vi "InitializeFileNoDig.vi"(0 "File Path":path=path "C:/Users/lbignell/Desktop/1 Ton Tank Experiment/Control Software/HDF5/Dummy2.h5", 1 "Thermocouple Location":string[](array[string])=["In Dark Box", "In Room"], 2 "Run Number":i32, 3 "VME Configuration":T1={"Module Description"=["Bridge", "TDC", "Scaler", "Hodoscope QDC ", "Other QDC", "Digitizer 1", "Digitizer 2", ""], "Module Model"=["V2718", "V775", "V830", "V965A", "V965A", "V1729A", "1729A", ""], "Module Address"=[0, 4026597376, 4026662912, 4026728448, 4026793984, 4026859520, 4026925056]} {"Module Address" format="%.0x"}, 4 "Trigger Bit Descriptions":string[](array[string])=["TrigA", "TrigB", "TrigC", "TrigD"], 5 "error in":errorcluster, 6 "Scaler Info":T3={"Chanel Description"=["H0", "H1", "H2", "H3", "H4", "H5", "TrigA", "TrigB", "TrigC", "TrigD", "Ch0", "Ch1", "Ch2", "Ch3", "Ch4", "Ch5", "Ch6", "Ch7"], "Only Hodo?"=[TRUE, TRUE, TRUE, TRUE, TRUE, TRUE, TRUE, TRUE, FALSE, FALSE, FALSE, FALSE, FALSE, FALSE, FALSE, FALSE, FALSE, FALSE]}, 7 "Optional Comments":string, 9 "Material in Tank":string(combo), 10 "Run Type":string(combo), 11 "TDC Info":T3={"Chanel Description"=["H0", "H1", "H2", "H3", "H4", "H5", "TrigA", "TrigB", "TrigC", "TrigD"], "Only Hodo?"=[TRUE, TRUE, TRUE, TRUE, TRUE, TRUE, TRUE, TRUE, FALSE, FALSE]}, 12 "QDC Info":T3={"Chanel Description"=["H0", "H1", "H2", "H3", "H4", "H5"], "Only Hodo?"=[TRUE, TRUE, TRUE, TRUE, TRUE, TRUE]}) -> (14 "File Handle":T2=16777216 format="%.0x", 19 "error out":errorcluster)   [LabVIEW 2014]
uses:
  <vilib>/addons/h5labview2/base/hid_t.ctl
  <vilib>/addons/h5labview2/file/H5Fmode.ctl
  <vilib>/addons/h5labview2/base/lib_path.vi
  <vilib>/addons/h5labview2/base/H5Equery.vi
  DatasetNames.vi
  <vilib>/addons/h5labview2/dataset/H5Dwrite.llb/H5Dwrite.xnode
  <vilib>/addons/h5labview2/file/H5F.lvlib
  <vilib>/addons/h5labview2/group/H5G.lvlib
  <vilib>/addons/h5labview2/props/H5P.lvlib
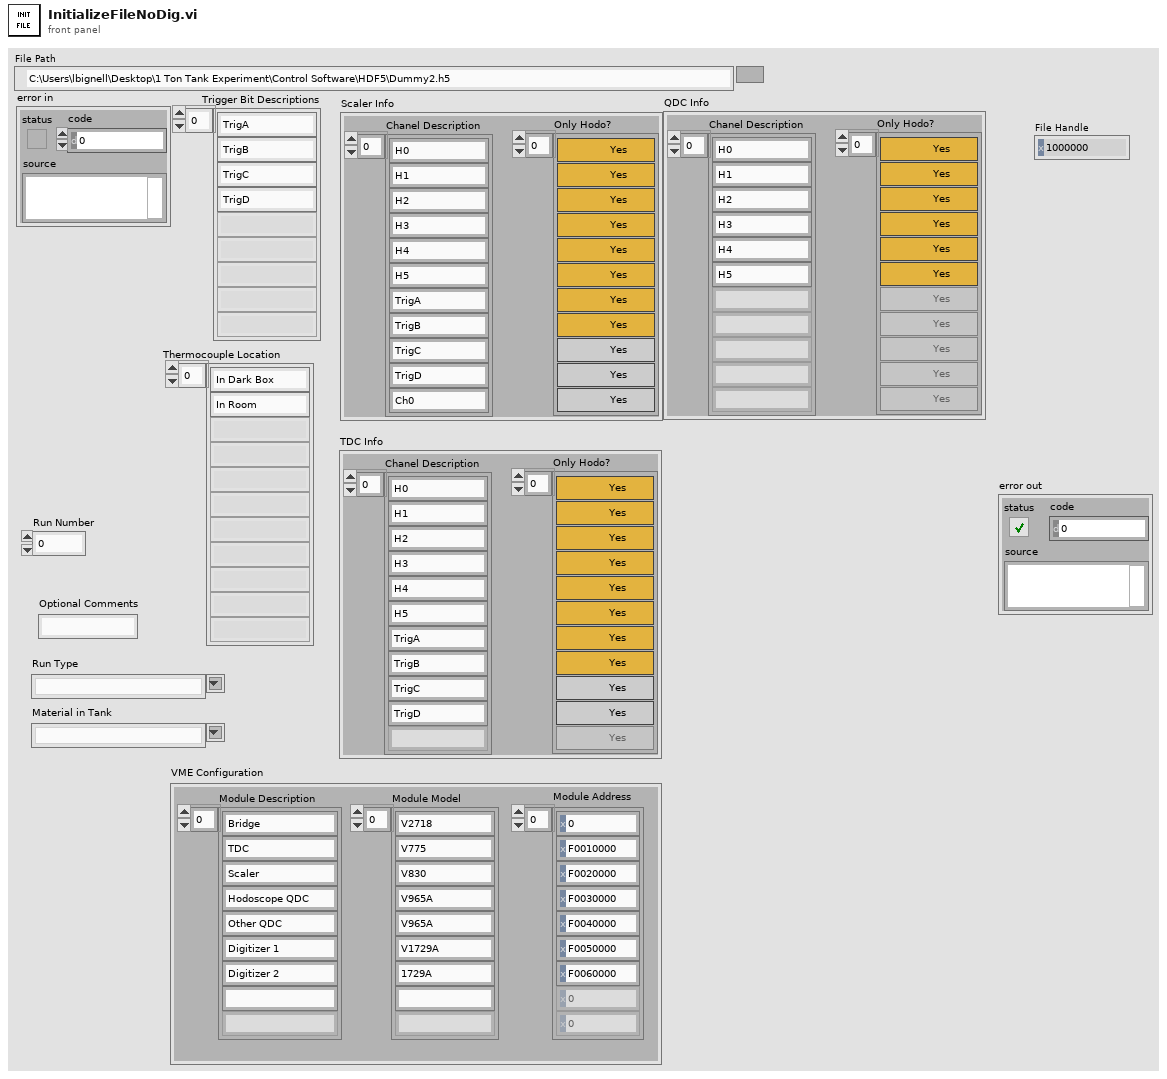
[diagram p1: front panel]
types:
  T1 = cluster{"Module Description":string[], "Module Model":string[], "Module Address":u32[]}
  T2 = typedef "hid_t.ctl" = i32
  T3 = cluster{"Chanel Description":string[], "Only Hodo?":bool[]}
  T4 = typedef "H5F.lvlib/H5Fmode.ctl" = enum16{"read-only", "read-write", "overwrite", "create new", "open or create"}
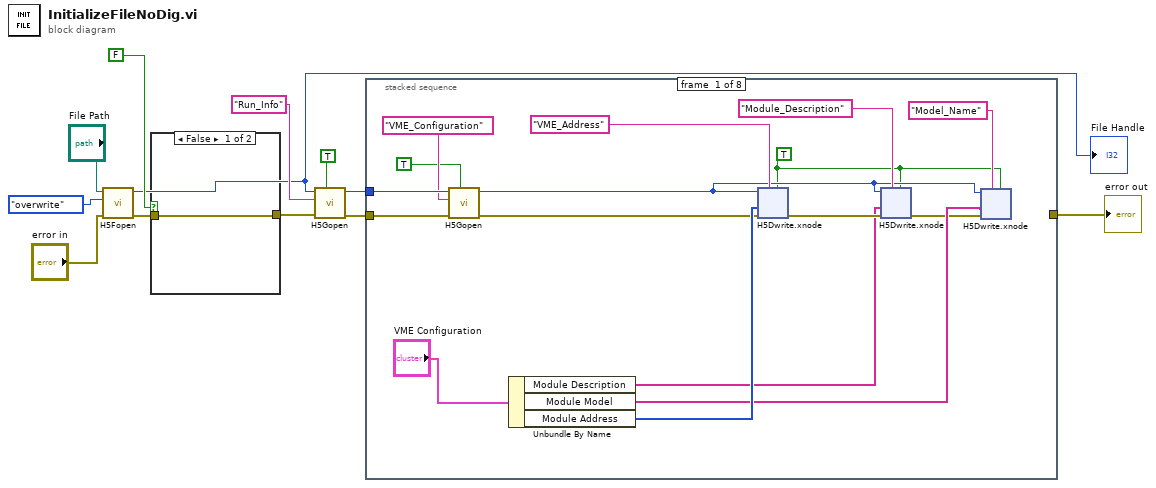
[diagram p0: block diagram]
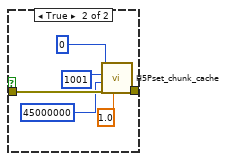
[diagram p2: hidden frame]
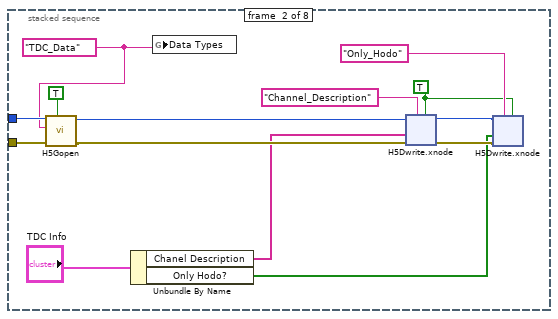
[diagram p3: hidden frame]
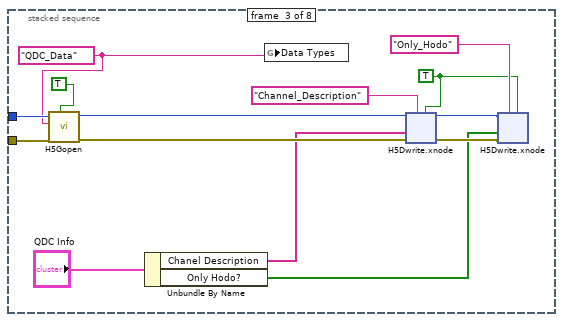
[diagram p4: hidden frame]
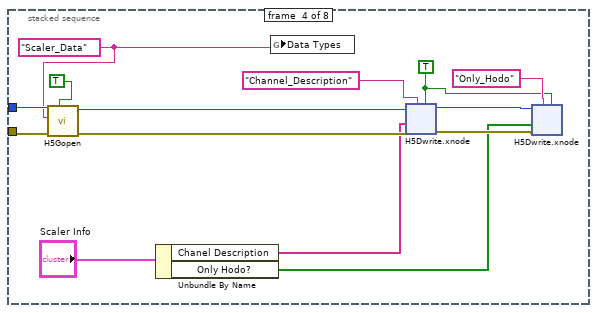
[diagram p5: hidden frame]
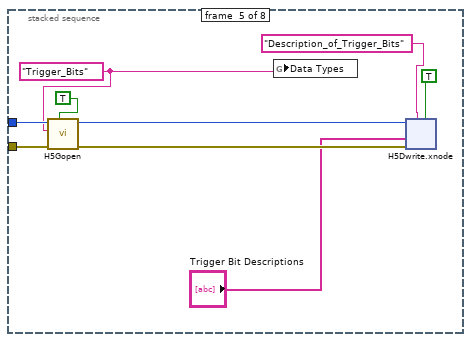
[diagram p6: hidden frame]
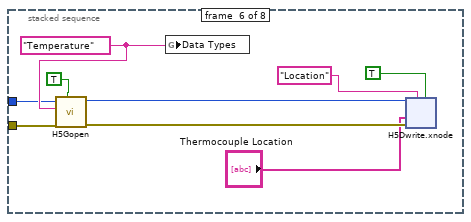
[diagram p7: hidden frame]
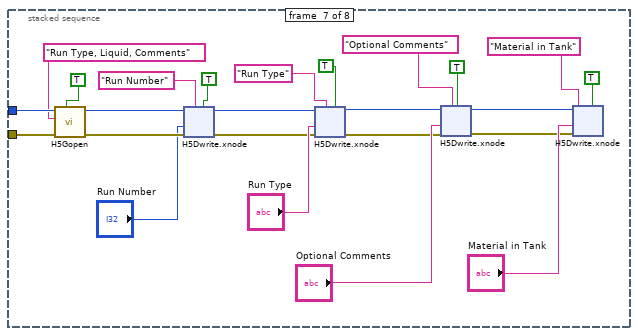
[diagram p8: hidden frame]
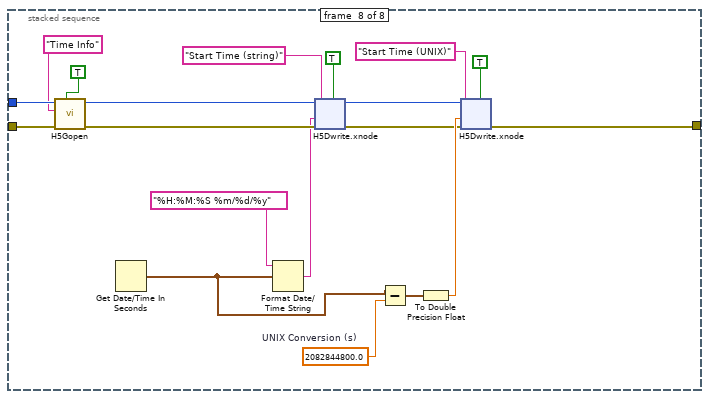
[diagram p9: hidden frame]
diagram:
  n1 = call <vilib>:"H5Fopen.vi"("error in (no error)"="error in", "mode (read-only)"=H5Fmode."overwrite", "path"="File Path") -> ("error out"=w4:errorcluster, "ref out"=w1:T2)  [unwired: 7 in]
  "File Handle" <- w1
  n2 = case shown="False" FALSE {
    tunnel: w4 -> [w13 w19]
    tunnel: [w13 w18] -> w3
    frame False {
    }
    frame True {
      n3 = call <vilib>:"H5Pset_chunk_cache.vi"("w0"=1.0, "error in (no error)"=w19, "nbytes"=u32 45000000, "nslots"=u32 1001, "prop in"=T2 0) -> ("error out"=w18:errorcluster)  [unwired: 5 in, 1 out]
    }
  }
  n4 = call <vilib>:"H5Gopen.vi"("create? (F)"=TRUE, "error in (no error)"=w3, "name"="Run_Info", "ref in"=w1) -> ("error out"=w7:errorcluster, "group out"=w8:T2)  [unwired: 6 in]
  n5 = stacked-sequence {
    tunnel: w8 -> [w31 w100 w151 w201 w247 w268 w316 w407]
    tunnel: w7 -> [w32 w102 w152 w202 w246 w274 w317 w408]
    tunnel: [_ _ _ _ _ _ _ w390] -> w6
    frame #0 {
      w21 = TRUE ("replace? (F)")
      n6 = call <vilib>:"H5Gopen.vi"("create? (F)"=TRUE, "error in (no error)"=w32, "name"="VME_Configuration" ("attrib name"), "ref in"=w31) -> ("error out"=w29:errorcluster, "group out"=w25:T2)  [unwired: 6 in]
      n7 = Unbundle By Name("VME Configuration") -> ("Module Description"=w26:string[], "Module Model"=w23:string[], "Module Address"=w33:u32[])
      n8 = xnode "H5Dwrite.xnode"("replace? (F)"=w21, "dataset name"="VME_Address" ("attrib name"), "error in (no error)"=w29, "data"=w33, "ref in"=w25) -> ("error out"=w27:errorcluster)  [unwired: 2 in, 2 out]
      n9 = xnode "H5Dwrite.xnode"("replace? (F)"=w21, "dataset name"="Module_Description" ("attrib name"), "error in (no error)"=w27, "data"=w26, "ref in"=w25) -> ("error out"=w22:errorcluster)  [unwired: 2 in, 2 out]
      n10 = xnode "H5Dwrite.xnode"("replace? (F)"=w21, "dataset name"="Model_Name" ("attrib name"), "error in (no error)"=w22, "data"=w23, "ref in"=w25) -> ()  [unwired: 2 in, 3 out]
    }
    frame #1 {
      w91 = TRUE ("replace? (F)")
      w99 = "TDC_Data" ("Combo Box")
      n11 = call <vilib>:"H5Gopen.vi"("create? (F)"=TRUE, "error in (no error)"=w102, "name"=w99, "ref in"=w100) -> ("error out"=w101:errorcluster, "group out"=w96:T2)  [unwired: 6 in]
      n12 = Unbundle By Name("TDC Info") -> ("Chanel Description"=w95:string[], "Only Hodo?"=w90:bool[])
      n13 = global write "DatasetNames.vi" "Data Types"(w99) -> ()
      n14 = xnode "H5Dwrite.xnode"("replace? (F)"=w91, "dataset name"="Channel_Description" ("attrib name"), "error in (no error)"=w101, "data"=w95, "ref in"=w96) -> ("error out"=w94:errorcluster, "ref out"=w93:i32)  [unwired: 2 in, 1 out]
      n15 = xnode "H5Dwrite.xnode"("replace? (F)"=w91, "dataset name"="Only_Hodo" ("attrib name"), "error in (no error)"=w94, "data"=w90, "ref in"=w93) -> ()  [unwired: 2 in, 3 out]
    }
    frame #2 {
      w141 = TRUE ("replace? (F)")
      w148 = "QDC_Data" ("Combo Box")
      n16 = call <vilib>:"H5Gopen.vi"("create? (F)"=TRUE ("replace? (F)"), "error in (no error)"=w152, "name"=w148, "ref in"=w151) -> ("error out"=w149:errorcluster, "group out"=w150:T2)  [unwired: 6 in]
      n17 = Unbundle By Name("QDC Info") -> ("Chanel Description"=w145:string[], "Only Hodo?"=w140:bool[])
      n18 = global write "DatasetNames.vi" "Data Types"(w148) -> ()
      n19 = xnode "H5Dwrite.xnode"("replace? (F)"=w141, "dataset name"="Channel_Description" ("attrib name"), "error in (no error)"=w149, "data"=w145, "ref in"=w150) -> ("error out"=w144:errorcluster, "ref out"=w143:i32)  [unwired: 2 in, 1 out]
      n20 = xnode "H5Dwrite.xnode"("replace? (F)"=w141, "dataset name"="Only_Hodo" ("attrib name"), "error in (no error)"=w144, "data"=w140, "ref in"=w143) -> ()  [unwired: 2 in, 3 out]
    }
    frame #3 {
      w190 = TRUE ("replace? (F)")
      w198 = "Scaler_Data" ("Combo Box")
      n21 = call <vilib>:"H5Gopen.vi"("create? (F)"=TRUE, "error in (no error)"=w202, "name"=w198, "ref in"=w201) -> ("error out"=w199:errorcluster, "group out"=w200:T2)  [unwired: 6 in]
      n22 = Unbundle By Name("Scaler Info") -> ("Chanel Description"=w195:string[], "Only Hodo?"=w191:bool[])
      n23 = global write "DatasetNames.vi" "Data Types"(w198) -> ()
      n24 = xnode "H5Dwrite.xnode"("replace? (F)"=w190, "dataset name"="Channel_Description" ("attrib name"), "error in (no error)"=w199, "data"=w195, "ref in"=w200) -> ("error out"=w194:errorcluster, "ref out"=w193:i32)  [unwired: 2 in, 1 out]
      n25 = xnode "H5Dwrite.xnode"("replace? (F)"=w190, "dataset name"="Only_Hodo" ("attrib name"), "error in (no error)"=w194, "data"=w191, "ref in"=w193) -> ()  [unwired: 2 in, 3 out]
    }
    frame #4 {
      w243 = "Trigger_Bits" ("Combo Box")
      n26 = call <vilib>:"H5Gopen.vi"("create? (F)"=TRUE ("replace? (F)"), "error in (no error)"=w246, "name"=w243, "ref in"=w247) -> ("error out"=w245:errorcluster, "group out"=w244:T2)  [unwired: 6 in]
      n27 = global write "DatasetNames.vi" "Data Types"(w243) -> ()
      n28 = xnode "H5Dwrite.xnode"("replace? (F)"=TRUE, "dataset name"="Description_of_Trigger_Bits" ("attrib name"), "error in (no error)"=w245, "data"="Trigger Bit Descriptions", "ref in"=w244) -> ()  [unwired: 2 in, 3 out]
    }
    frame #5 {
      w272 = "Temperature" ("Combo Box")
      n29 = call <vilib>:"H5Gopen.vi"("create? (F)"=TRUE ("replace? (F)"), "error in (no error)"=w274, "name"=w272, "ref in"=w268) -> ("error out"=w273:errorcluster, "group out"=w267:T2)  [unwired: 6 in]
      n30 = global write "DatasetNames.vi" "Data Types"(w272) -> ()
      n31 = xnode "H5Dwrite.xnode"("replace? (F)"=TRUE, "dataset name"="Location" ("attrib name"), "error in (no error)"=w273, "data"="Thermocouple Location", "ref in"=w267) -> ()  [unwired: 2 in, 3 out]
    }
    frame #6 {
      n32 = call <vilib>:"H5Gopen.vi"("create? (F)"=TRUE, "error in (no error)"=w317, "name"="Run Type, Liquid, Comments", "ref in"=w316) -> ("error out"=w297:errorcluster, "group out"=w299:T2)  [unwired: 6 in]
      n33 = xnode "H5Dwrite.xnode"("replace? (F)"=TRUE, "dataset name"="Run Number", "error in (no error)"=w297, "data"="Run Number", "ref in"=w299) -> ("error out"=w298:errorcluster, "ref out"=w300:i32)  [unwired: 2 in, 1 out]
      n34 = xnode "H5Dwrite.xnode"("replace? (F)"=TRUE, "dataset name"="Run Type", "error in (no error)"=w298, "data"="Run Type", "ref in"=w300) -> ("error out"=w309:errorcluster, "ref out"=w308:i32)  [unwired: 2 in, 1 out]
      n35 = xnode "H5Dwrite.xnode"("replace? (F)"=TRUE, "dataset name"="Optional Comments", "error in (no error)"=w309, "data"="Optional Comments", "ref in"=w308) -> ("error out"=w304:errorcluster, "ref out"=w305:i32)  [unwired: 2 in, 1 out]
      n36 = xnode "H5Dwrite.xnode"("replace? (F)"=TRUE, "dataset name"="Material in Tank", "error in (no error)"=w304, "data"="Material in Tank", "ref in"=w305) -> ()  [unwired: 2 in, 3 out]
    }
    frame #7 {
      w399 = 2082844800.0  # UNIX Conversion (s)
      n37 = call <vilib>:"H5Gopen.vi"("create? (F)"=TRUE, "error in (no error)"=w408, "name"="Time Info", "ref in"=w407) -> ("error out"=w403:errorcluster, "group out"=w404:T2)  [unwired: 6 in]
      n38 = Get Date/Time In Seconds() -> (seconds since 1Jan1904=w398:timestamp)
      n39 = Format Date/Time String(time format string (%c)="%H:%M:%S %m/%d/%y", seconds (now)=w398) -> (date/time string=w400:string)  [unwired: 1 in]
      n40 = xnode "H5Dwrite.xnode"("replace? (F)"=TRUE, "dataset name"="Start Time (string)", "error in (no error)"=w403, "data"=w400, "ref in"=w404) -> ("error out"=w394:errorcluster, "ref out"=w395:i32)  [unwired: 2 in, 1 out]
      n41 = Subtract(x=w398, y=w399) -> (x-y=w397:timestamp)
      n42 = To Double Precision Float(number=w397) -> (double precision float=w396:dbl)
      n43 = xnode "H5Dwrite.xnode"("replace? (F)"=TRUE, "dataset name"="Start Time (UNIX)", "error in (no error)"=w394, "data"=w396, "ref in"=w395) -> ("error out"=w390:errorcluster)  [unwired: 2 in, 2 out]
    }
  }
  "error out" <- w6
